vi "dfd_DFXP_DFXP to Extended (scaler)64bits.vi"(11 "Value in":T1={"value"=0, "wl"=0, "iwl"=0, "Signed"=TRUE} {"value" format="%.0x"}) -> (3 "Ext":ext)   [LabVIEW 2017, in "NI_DigFilter_FXP.lvlib"]
uses:
  <vilib>/addons/Digital Filter Design/NI_DigFilter_FXP.lvlib
  <vilib>/addons/Digital Filter Design/_Objects.llb/dfd_DFXP Data Type (scaler).ctl
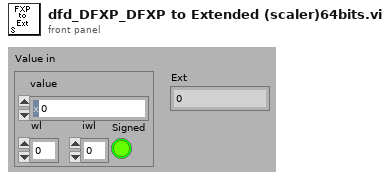
[diagram p1: front panel]
types:
  T1 = typedef "dfd_DFXP Data Type (scaler).ctl" = cluster{"value":i64, "wl":i16, "iwl":i16, "Signed":bool}
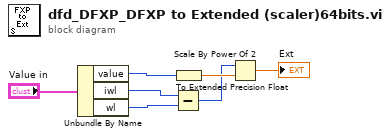
[diagram p0: block diagram]
diagram:
  n1 = Unbundle By Name("Value in") -> ("value"=w6:i64, "iwl"=w4:i16, "wl"=w5:i16)
  n2 = Subtract(x=w4, y=w5) -> (x-y=w2:i16)
  n3 = To Extended Precision Float(1:w6) -> (0:w3:ext)
  n4 = Scale By Power Of 2(n=w2, x=w3) -> (x*2^n=→"Ext":ext)
